vi "rad_ImageVersionDialog.vi"(1 "ShowUpgradeButton":bool, 2 "Message":string) -> ()   [LabVIEW 2013]
uses:
  rad_Globals.vi
  <vilib>/Platform/browser.llb/Open URL in Default Browser (string).vi
panel:
  in  "GetNewVersion":bool
  in  "OK":bool
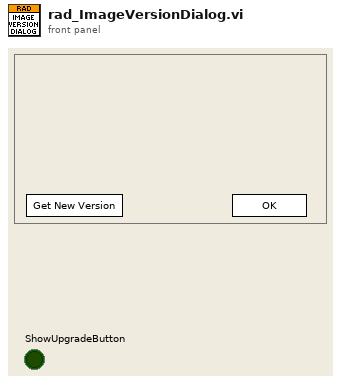
[diagram p1: front panel]
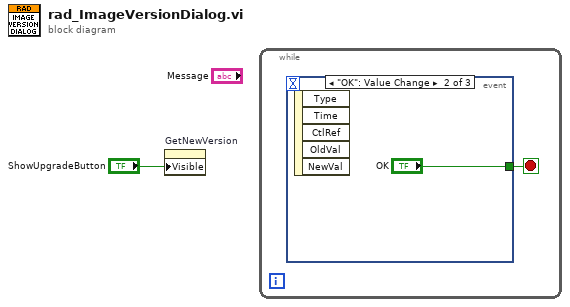
[diagram p0: block diagram]
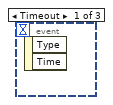
[diagram p2: hidden frame]
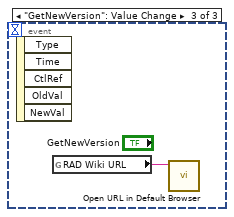
[diagram p3: hidden frame]
diagram:
  n1 = property on="GetNewVersion" class="Bool"("Visible"="ShowUpgradeButton") -> ()  [unwired: 2 in, 2 out]
  n2 = while {
    stop <- w2 stop-if-true
    n3 = event shown="[1] \"OK\": Value Change" {
      selector: _ -> [_ _ _]
      dyn-events: _ -> [_ _ _]
      timeout: _ -> [_ _ _]
      tunnel: [_ "OK" _] -> w2
      event Timeout {
        n4 = event-data() -> ()  [unwired: 1 in, 2 out]
      }
      event "OK": Value Change {
        n5 = event-data() -> ()  [unwired: 1 in, 5 out]
      }
      event "GetNewVersion": Value Change {
        n6 = event-data() -> ()  [unwired: 1 in, 5 out]
        n7 = global read "rad_Globals.vi" "RAD Wiki URL"() -> (w4:string)
        n8 = call-poly <vilib>:"Open URL in Default Browser.vi"("URL"=w4) -> ()  [unwired: 5 in, 2 out]
      }
    }
  }
